vi "test Camera Read N Images from Buffer.vi"(11 "Test Camera in":refnum<class "Test Camera.lvclass">) -> (0 "error out":errorcluster, 3 "Test Camera out":refnum<class "Test Camera.lvclass">)   [LabVIEW 2024, in "Test Camera.lvclass"]
uses:
  Test Camera.lvclass
  C:/Program Files/National Instruments/LabVIEW 2025/vi.lib/Astemes/LUnit/Test Case.lvclass
  Source/Configure Strategies/IMAQdx Strategies/Continuous Acquisition/IMAQdx Triggered Continuous Acquisition.lvclass
  D:/git/HAL/Source/Interfaces/IConfigure/IConfigure.lvclass
  Source/Config from JSON/Config from JSON.lvclass
  D:/git/HAL/Source/Interfaces/IConfiguration/IConfiguration.lvclass
  Source/Camera/Camera.lvclass
  <vilib>/Astemes/LUnit/Test Case.lvclass/Test Case.ctl
  <vilib>/Astemes/LUnit/Test Case.lvclass
  Source/Typedefs/Generic Image/Generic Image.lvclass
panel:
  out "iter time":dbl
  out "Intensity Graph":u16[][](graph)
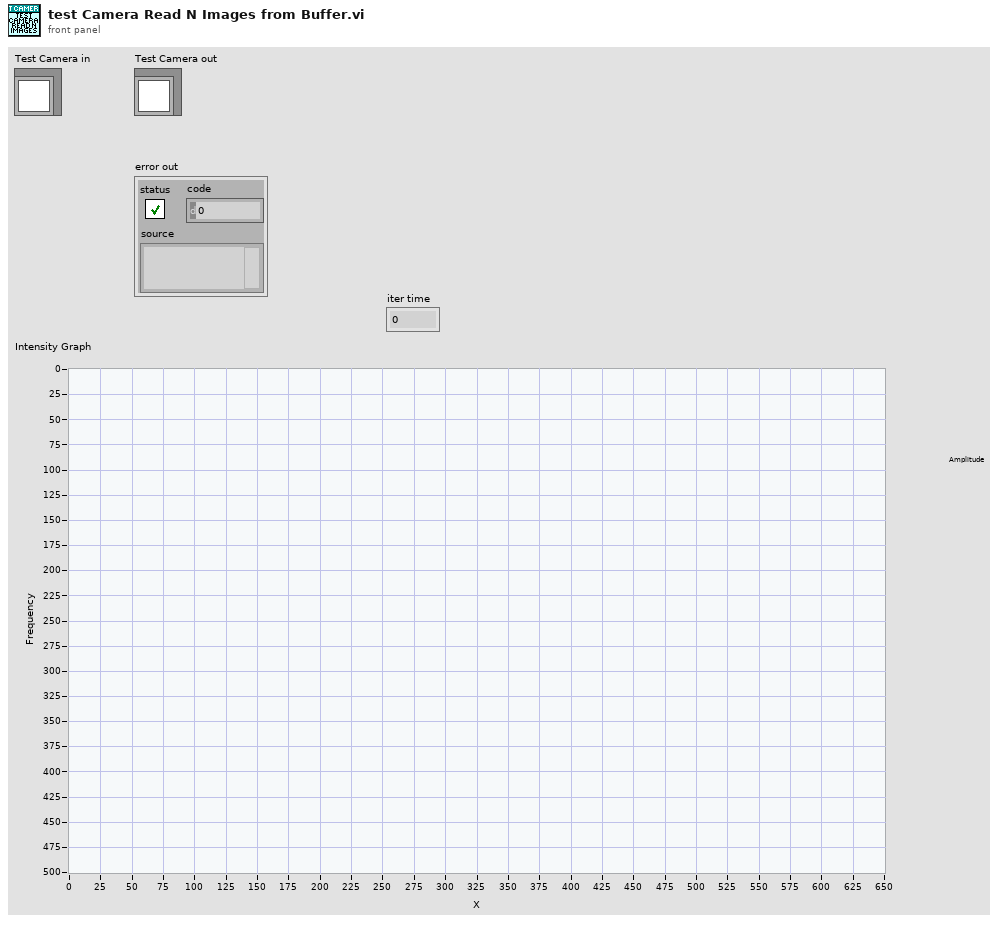
[diagram p1: front panel]
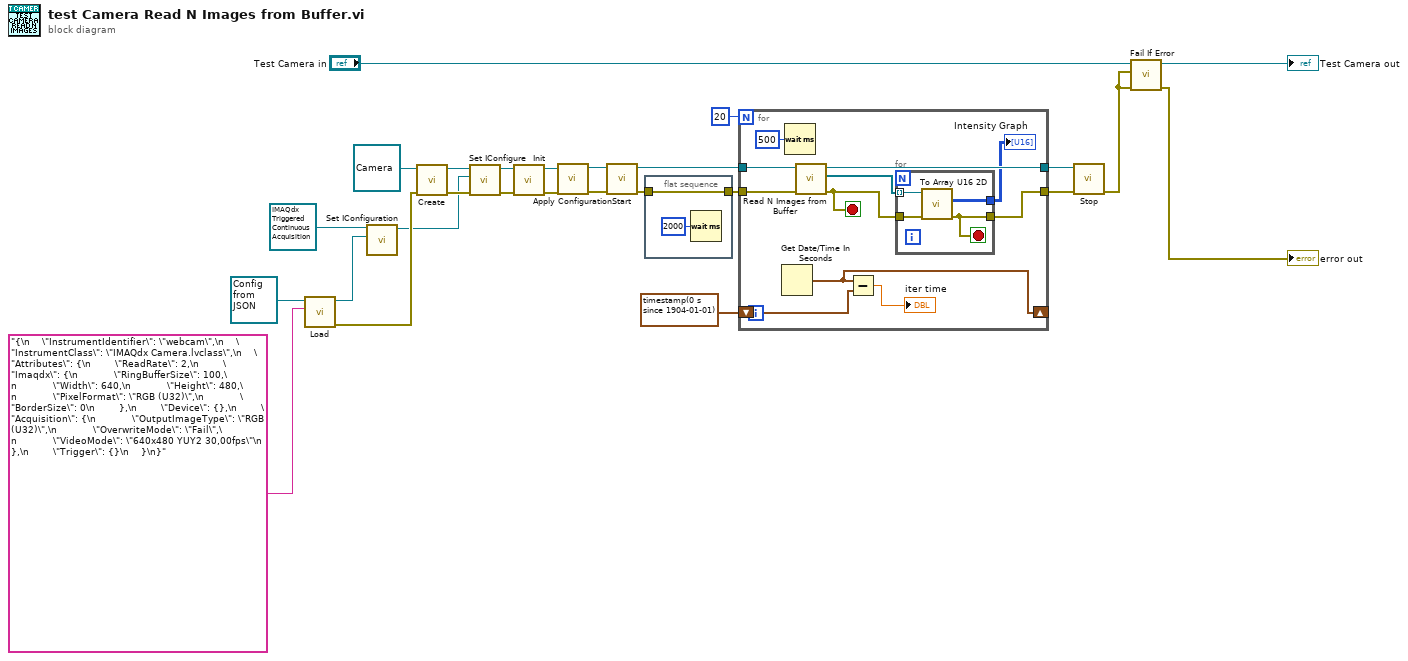
[diagram p0: block diagram]
diagram:
  n1 = call-dynamic "Load.vi"("Source"="{\n    \"InstrumentIdentifier\": \"webcam\",\n    \"InstrumentClass\": \"IMAQdx Camera.lvclass\",\n    \"Attributes\": {\n        \"ReadRate\": 2,\n        \"Imaqdx\": {\n            \"RingBufferSize\": 100,\n            \"Width\": 640,\n            \"Height\": 480,\n            \"PixelFormat\": \"RGB (U32)\",\n            \"BorderSize\": 0\n        },\n        \"Device\": {},\n        \"Acquisition\": {\n            \"OutputImageType\": \"RGB (U32)\",\n            \"OverwriteMode\": \"Fail\",\n            \"VideoMode\": \"640x480 YUY2 30,00fps\"\n        },\n        \"Trigger\": {}\n    }\n}", "Config From JSON in"=refnum<class "Config from JSON.lvclass"> refnum ("Config from JSON.lvclass")) -> ("error out"=w17:errorcluster, "Config From JSON out"=w18:refnum<class "Config from JSON.lvclass">)  [unwired: 8 in]
  n2 = call-dynamic "Set IConfiguration.vi"("IConfiguration"=w18, "IMAQdx Base Configure Strategy in"=refnum<class "IMAQdx Triggered Continuous Acquisition.lvclass"> refnum ("IMAQdx Triggered Continuous Acquisition.lvclass")) -> ("IMAQdx Base Configure Strategy out"=w16:refnum<class "IMAQdx Triggered Continuous Acquisition.lvclass">)  [unwired: 9 in]
  n3 = call-dynamic "Create.vi"("Error In"=w17, "reference in"=refnum<class "Camera.lvclass"> refnum ("Camera")) -> ("Error Out"=w23:errorcluster, "reference out"=w22:refnum<class "Camera.lvclass">)  [unwired: 8 in]
  n4 = call-dynamic "Set IConfigure.vi"("Error In"=w23, "IConfigure"=w16, "reference in"=w22) -> ("Error Out"=w15:errorcluster, "reference out"=w13:refnum<class "Camera.lvclass">)  [unwired: 7 in]
  n5 = call-dynamic "Init.vi"("Error In"=w15, "reference in"=w13) -> ("Error Out"=w14:errorcluster, "reference out"=w12:refnum<class "Camera.lvclass">)  [unwired: 8 in]
  n6 = call-dynamic "Apply Configuration.vi"("Error In"=w14, "reference in"=w12) -> ("Error Out"=w11:errorcluster, "reference out"=w10:refnum<class "Camera.lvclass">)  [unwired: 8 in]
  n7 = call-dynamic "Start.vi"("Error In"=w11, "reference in"=w10) -> ("Error Out"=w5:errorcluster, "reference out"=w9:refnum<class "Camera.lvclass">)  [unwired: 8 in]
  n8 = flat-sequence {
    tunnel: w5 -> [w27]
    tunnel: [w27] -> w4
    frame #0 {
      n9 = Wait (ms)(milliseconds to wait=u32 2000) -> ()  [unwired: 1 out]
    }
  }
  n10 = for {
    N: 20 -> [_]
    tunnel: w9 -> [w38]
    tunnel: w4 -> [w39]
    tunnel: [w37] -> w7
    tunnel: [w34] -> w8
    shift-right: [w30] -> _
    shift-left: timestamp(0 s since 1904-01-01) -> [w31]
    stop <- w35 stop-if-true
    n11 = Get Date/Time In Seconds() -> (seconds since 1Jan1904=w30:timestamp)
    n12 = Wait (ms)(milliseconds to wait=u32 500) -> ()  [unwired: 1 out]
    n13 = call-dynamic "Read N Images from Buffer.vi"("Error In"=w39, "reference in"=w38) -> ("Error Out"=w35:errorcluster, "images"=w32:refnum<class "Generic Image.lvclass">[], "reference out"=w37:refnum<class "Camera.lvclass">)  [unwired: 7 in]
    n14 = Subtract(x=w30, y=w31) -> (x-y=→"iter time":dbl)
    n15 = for {
      tunnel: [w42] -> w33
      tunnel: w35 -> [w43]
      tunnel: [w41] -> w34
      tunnel: w32 -> [w40] mode=indexing
      stop <- w41 stop-if-true
      n16 = call "To Array U16 2D.vi"("error in"=w43, "Generic Image in"=w40) -> ("error out"=w41:errorcluster, "U16"=w42:u16[][])  [unwired: 6 in, 2 out]
    }
    "Intensity Graph" <- w33
  }
  n17 = call-dynamic "Stop.vi"("Error In"=w8, "reference in"=w7) -> ("Error Out"=w6:errorcluster)  [unwired: 8 in, 1 out]
  n18 = call <vilib>:"Fail If Error.vi"("error in (no error)"=w6, "Assert error"=w6, "LUnit Test Case In"="Test Camera in") -> ("error out"=→"error out":errorcluster, "LUnit Test Case Out"=→"Test Camera out":refnum<class "Test Camera.lvclass">)  [unwired: 7 in]
